vi "Monitor.vi"(7 "PV name":string, 8 "error in":errorcluster, 11 "Client in":refnum<class "Client.lvclass">) -> (0 "error out":errorcluster, 2 "subscription":refnum<class "Subscription.lvclass">, 3 "Client out":refnum<class "Client.lvclass">)   [LabVIEW 2020, in "PV Access.lvlib" / "PVA Client.lvlib" / "Client.lvclass"]
doc: "Monitor a PV and create a new subscription.\n\nWire the <B>subscription</B> into a while loop and retrieve new values with <B>Next Value.vim</B>."
uses:
  Client.lvclass
  Subscription/Subscription.lvclass
  Client.lvclass/Client.ctl
  PV Access.lvlib
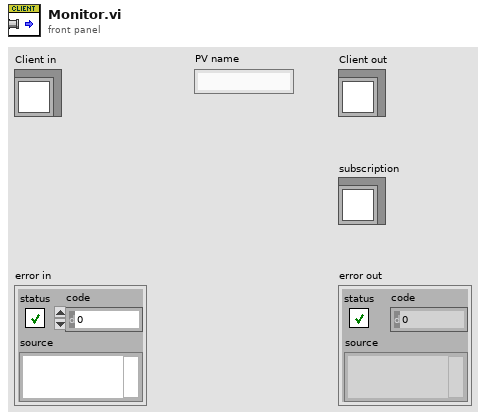
[diagram p1: front panel]
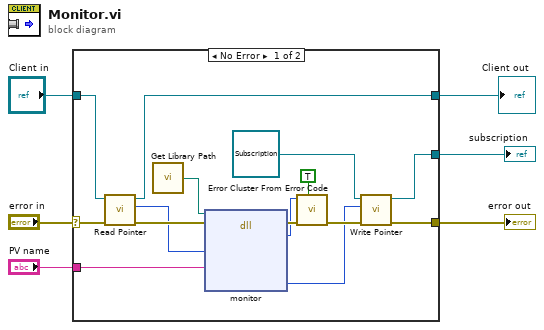
[diagram p0: block diagram]
diagram:
  n1 = case shown="No Error" "error in" {
    selector: "error in" -> [w21 w23]
    tunnel: [w11 w23] -> w3
    tunnel: [w12 w22] -> w2
    tunnel: "Client in" -> [w17 w22]
    tunnel: "PV name" -> [w18 _]
    tunnel: [w7 _] -> w1
    frame No Error {
      n2 = call-dynamic "Read Pointer.vi"("error in (no error)"=w21, "Pointer Base in"=w17) -> ("error out"=w20:errorcluster, "Pointer"=w19:i64, "Pointer Base out"=w12:refnum<class "Client.lvclass">)  [unwired: 7 in]
      n3 = call "Get Library Path.vi"() -> ("Path"=w16:path)  [unwired: 1 in]
      n4 = dll-call lib="?" fn="monitor"(path in=w16, error in=w20, "client"=w19, "pv_name"=w18) -> (error out=w14:errorcluster, "ret_code"=w13:i32, "subscription"=w9:i64)  [unwired: 4 in, 1 out]
      n5 = call <vilib>:"Error Cluster From Error Code.vi"("show call chain? (False)"=TRUE, "error in (no error)"=w14, "error code (0)"=w13) -> ("error out"=w10:errorcluster)  [unwired: 6 in]
      n6 = call-dynamic "Write Pointer.vi"("error in (no error)"=w10, "Pointer"=w9, "Pointer Base in"=refnum<class "Subscription.lvclass"> refnum ("Client.lvlib:Subscription.lvclass")) -> ("error out"=w11:errorcluster, "Pointer Base out"=w7:refnum<class "Subscription.lvclass">)  [unwired: 7 in]
    }
    frame Error {
    }
  }
  "error out" <- w3
  "Client out" <- w2
  "subscription" <- w1
